vi "create.vi"(8 "error in (no error)":errorcluster) -> (0 "error out":errorcluster, 3 "midi-callback-userevent out":refnum<class "midi-callback-userevent.lvclass">)   [LabVIEW 2020, in "midi-callback-userevent.lvclass"]
uses:
  midi-callback-userevent.lvclass
  midi-callback-userevent.lvclass/midi-callback-userevent.ctl
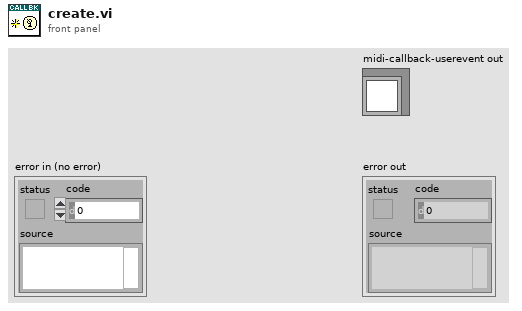
[diagram p1: front panel]
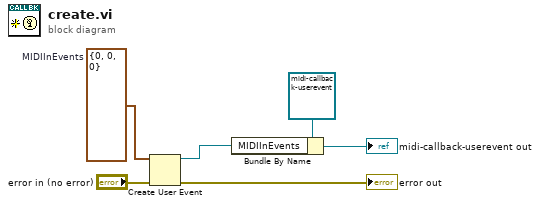
[diagram p0: block diagram]
diagram:
  w6 = cluster{"Status":i32, "Data1":i32, "Data2":i32} {"Status"=0, "Data1"=0, "Data2"=0}  # MIDIInEvents
  n1 = Create User Event(user event datatype=w6, error in="error in (no error)") -> (user event=w5:refnum<user-event>, error out=→"error out":errorcluster)
  n2 = Bundle By Name(cluster=refnum<class "midi-callback-userevent.lvclass"> refnum ("midi-callback-userevent out"), "MIDIInEvents"=w5) -> (→"midi-callback-userevent out":refnum<class "midi-callback-userevent.lvclass">)
